vi "Data_I2C.vi"() -> ()   [LabVIEW 2020, in "I2C Module.lvlib"]
uses:
  I2C Module.lvlib
panel:
  in  "dt":dbl
  out "Digital Waveform Graph":digitaldata(graph)
  in  "Stop":bool
  in  "Voltage":dbl=2.0 min=1.8 max=5.0 step=0.1
  in  "Data":string
  in  "Stop":bool
  out "I2C DATA":dbl[][](graph)
  in  "Address":u8 max=127 step=1 format="%x"
  in  "Start":bool
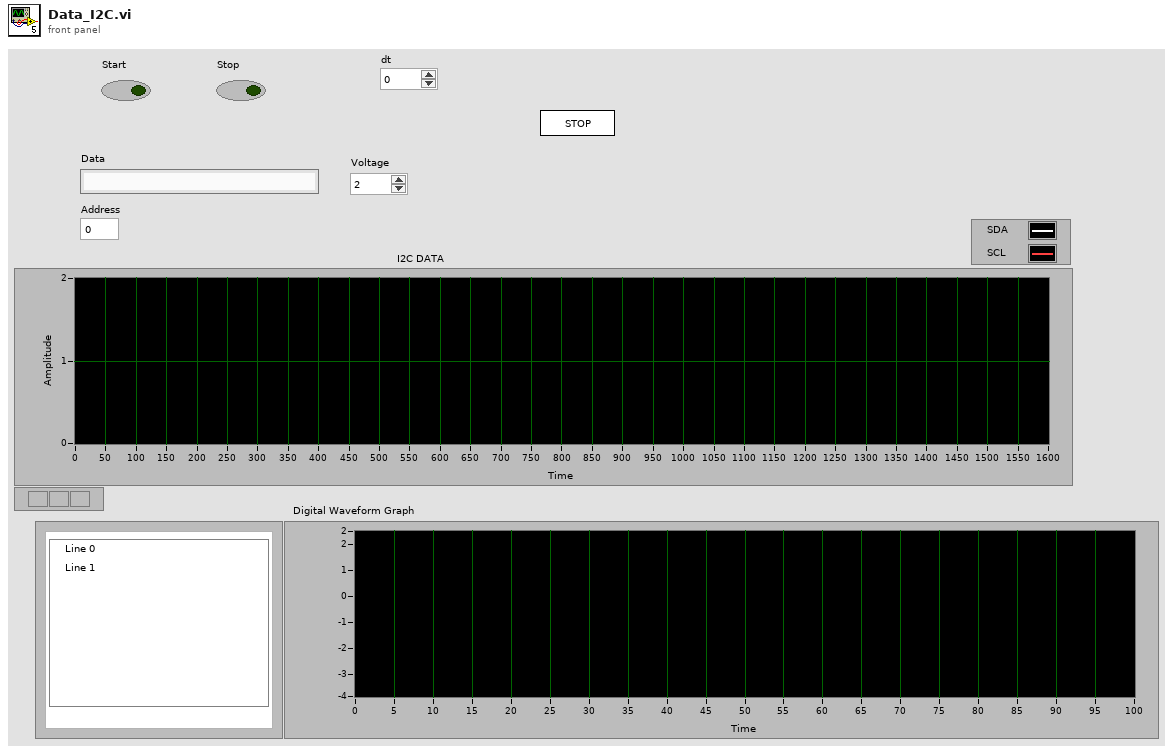
[diagram p1: front panel]
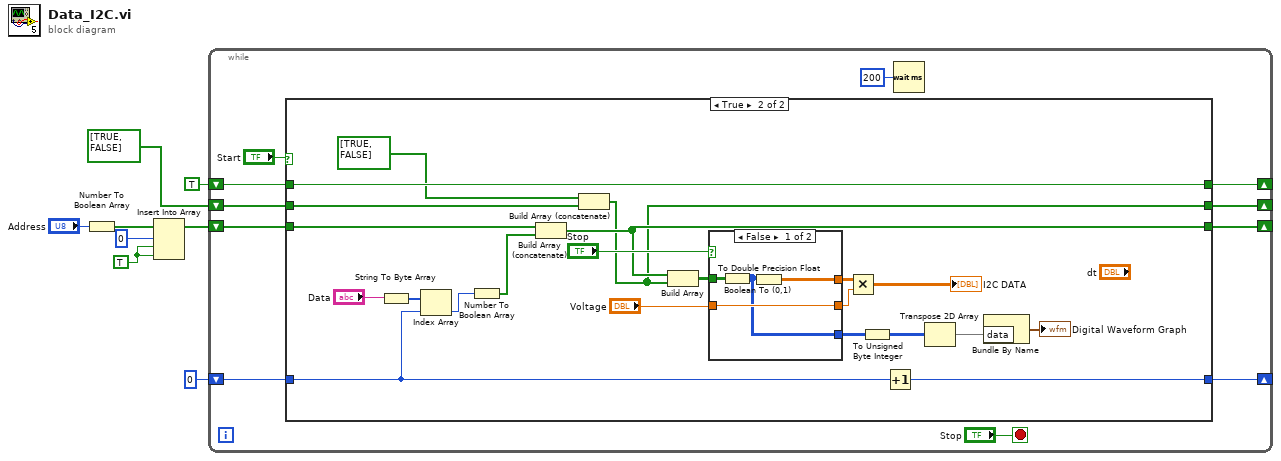
[diagram p0: block diagram]
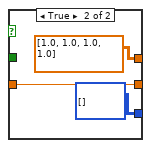
[diagram p3: hidden frame]
diagram:
  w5 = TRUE ("new element/subarray")
  n1 = Number To Boolean Array(number="Address") -> (Boolean array=w8:bool[])
  n2 = Insert Into Array(array=w8, index=0, new element #1=w5, new element #2=w5) -> (w4:bool[])
  n3 = while {
    shift-right: [w14] -> _
    shift-left: w4 -> [w17]
    shift-right: [w15] -> _
    shift-left: 0 -> [w16]
    shift-right: [w9] -> _
    shift-left: TRUE -> [w12]
    shift-right: [w11] -> _
    shift-left: bool[] [TRUE, FALSE] -> [w10]
    stop <- "Stop" stop-if-true
    n4 = case shown="True" "Start" {
      tunnel: [w22 w31] -> w14
      tunnel: w17 -> [w22 w44]
      tunnel: w16 -> [w23 w41]
      tunnel: [w23 w42] -> w15
      tunnel: w12 -> [w21 w37]
      tunnel: [w21 w37] -> w9
      tunnel: [w20 w30] -> w11
      tunnel: w10 -> [w20 w38]
      frame False {
      }
      frame True {
        n5 = String To Byte Array(string="Data") -> (unsigned byte array=w43:u8[])
        n6 = Index Array(array=w43, index=w41) -> (element=w40:u8)
        n7 = Number To Boolean Array(number=w40) -> (Boolean array=w39:bool[])
        n8 = Build Array (concatenate)(w44, w39) -> (w31:bool[])
        n9 = Build Array (concatenate)(bool[] [TRUE, FALSE], w38) -> (w30:bool[])
        n10 = Build Array(w31, w30) -> (w29:bool[][])
        n11 = case shown="False" "Stop" {
          tunnel: w29 -> [w49 _]
          tunnel: "Voltage" -> [w48 w51]
          tunnel: [w47 dbl[][] [[1.0, 1.0, 1.0, 1.0]]] -> w34
          tunnel: [w48 w51] -> w33
          tunnel: [w46 i16[][] []] -> w27
          frame False {
            n12 = Boolean To (0,1)(Boolean=w49) -> (0, 1=w46:i16[][])
            n13 = To Double Precision Float(number=w46) -> (double precision float=w47:dbl[][])
          }
          frame True {
          }
        }
        n14 = Multiply(x=w34, y=w33) -> (x*y=→"I2C DATA":dbl[][])
        n15 = To Unsigned Byte Integer(number=w27) -> (unsigned 8bit integer=w25:u8[][])
        n16 = Increment(x=w41) -> (x+1=w42:i32)
        n17 = Transpose 2D Array(2D array=w25) -> (transposed array=w24:u8[][])
        n18 = Bundle By Name("data"=w24) -> (→"Digital Waveform Graph":digitaldata)  [unwired: 1 in]
      }
    }
    n19 = Wait (ms)(milliseconds to wait=u32 200) -> ()  [unwired: 1 out]
  }
